vi "Set vim properties.vi"() -> ()   [LabVIEW 2018]
panel:
  out "error out":errorcluster
  out "All Files in Dir":path[](array[path])
  in  "Directory":path
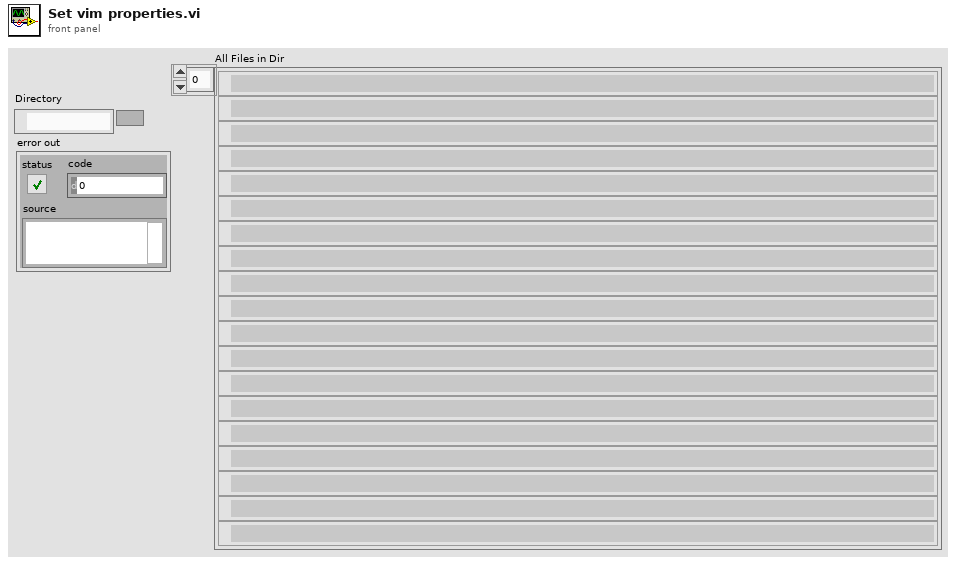
[diagram p1: front panel]
types:
  T1 = enum16{"Share clones between instances", "Preallocate clone for each instance"}
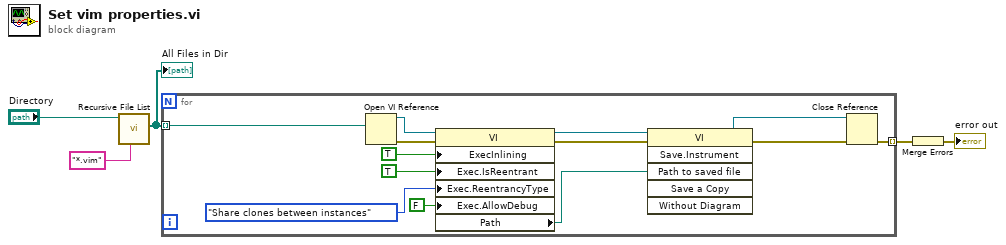
[diagram p0: block diagram]
diagram:
  n1 = call <vilib>:"Recursive File List.vi"("pattern"="*.vim", "Folder Path"="Directory") -> ("All Files in Dir"=w3:path[])  [unwired: 5 in, 4 out]
  "All Files in Dir" <- w3
  n2 = for {
    tunnel: w3 -> [w18] mode=indexing
    tunnel: [w10] -> w2 mode=indexing
    n3 = Open VI Reference(vi path=w18) -> (vi reference=w17:refnum<vi>, error out=w16:errorcluster)  [unwired: 5 in]
    n4 = property class="VI"(reference=w17, error in=w16, "ExecInlining"=TRUE ("Execution:Inline SubVI"), "Exec.IsReentrant"=TRUE ("Execution:Is Reentrant"), "Exec.ReentrancyType"=T1."Share clones between instances" ("Execution:Reentrancy Type"), "Exec.AllowDebug"=FALSE ("Execution:Allow Debugging")) -> (reference out=w8:refnum<vi>, error out=w11:errorcluster, "Path"=w6:path)
    n5 = invoke class="VI" method="Save.Instrument"(reference=w8, error in=w11, "Path to saved file"=w6) -> (reference out=w7:refnum<vi>, error out=w9:errorcluster)  [unwired: 3 in, 4 out]
    n6 = Close Reference(reference=w7, error in (no error)=w9) -> (error out=w10:errorcluster)
  }
  n7 = Merge Errors(w2) -> (→"error out":errorcluster)
